vi "PowerEnergyMeterInit.vi"(1 "错误输入（无错误）":errorcluster) -> (0 "错误输出":errorcluster)   [LabVIEW 2012]
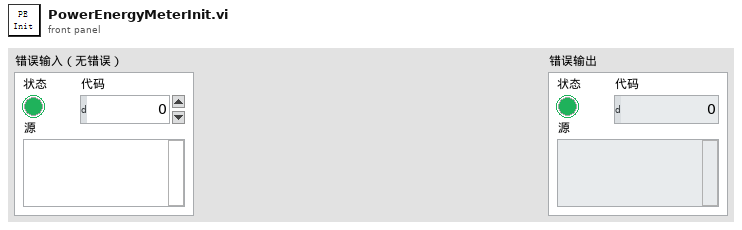
[diagram p1: front panel]
types:
  T1 = typedef "IMAQ Image.ctl" = refnum<image>
  T2 = cluster{"示波器":cluster{"Channel (0:Channel 1)":enum16{"Channel 1", "Channel 2", "Channel 3", "Channel 4"}, "电压范围":dbl, "触发电压":dbl, "时间范围":dbl, " 示波器VISA":refnum<visa-resource-name>}, "光谱仪":cluster{"Channel (0:Channel 1)":enum16{"Channel 1", "Channel 2", "Channel 3", "Channel 4"}, "电压范围":u64, "触发电压":u64, "时间范围":u64}, " 相机1":cluster{"曝光时间":i32, "模拟增益":i32, "控制套接字":i32, "IP 地址":string, " 采集套接字":i32, "  版本号":i32, "ImageData":T1, "  增益最大":i32, "  增益最小":i32, " 曝光最大":i32, " 曝光最小":i32, " 帧速":i32, " 同步切换":i32, "  曝光缩放":i32}, " 偏振仪":cluster{"波长范围":enum16{"可见光", "近红外"}, "电压范围":u64, "触发电压":u64, "时间范围":u64}, " 功率计":cluster{"通道":enum16{"Channel 1", "Channel 2"}, "工作波长":u64, "单位":u64, "时间范围":u64}, "能量计":cluster{"通道":enum16{"Channel 1", "Channel 2"}, "工作波长":u64, "单位":u64, "时间范围":u64}, "电机":cluster{"Channel (0:Channel 1)":enum16{"Channel 1", "Channel 2", "Channel 3", "Channel 4"}, "电压范围":u64, "触发电压":u64, "时间范围":u64}}
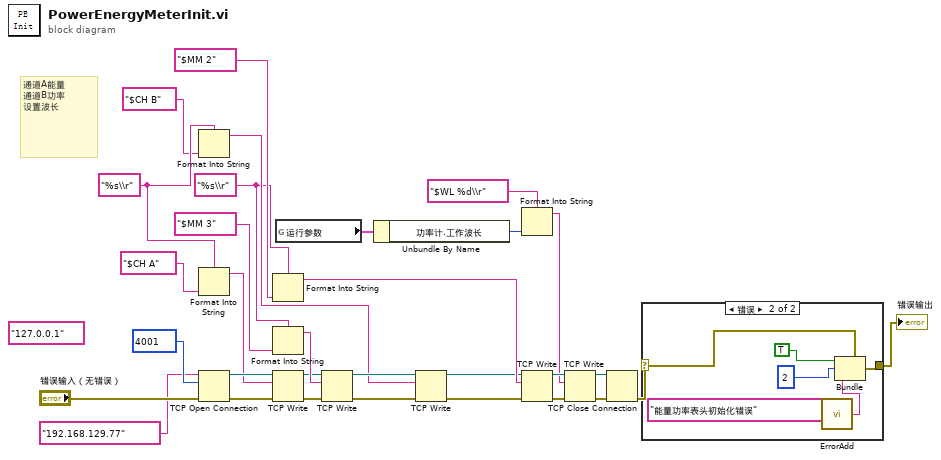
[diagram p0: block diagram]
diagram:
  (unwired) "127.0.0.1" ("地址")
  w20 = "%s\\r" ("格式字符串")
  w12 = "%s\\r" ("格式字符串")
  # "通道A能量\n通道B功率\n设置波长"
  n1 = Format Into String(format string=w20, "$CH B" ("输入 1")) -> (resulting string=w18:string)  [unwired: 2 in, 1 out]
  n2 = Format Into String(format string=w20, "$CH A" ("输入 1")) -> (resulting string=w26:string)  [unwired: 2 in, 1 out]
  n3 = TCP Open Connection(address="192.168.129.77" ("地址"), remote port or service name=u16 4001 ("远程端口或服务名称"), error in (no error)="错误输入（无错误）") -> (connection ID=w27:refnum<k5>, error out=w25:errorcluster)  [unwired: 2 in]
  n4 = Format Into String(format string=w12, "$MM 2" ("输入 1")) -> (resulting string=w15:string)  [unwired: 2 in, 1 out]
  n5 = Format Into String(format string=w12, "$MM 3" ("输入 1")) -> (resulting string=w29:string)  [unwired: 2 in, 1 out]
  n6 = TCP Write(connection ID=w27, data in=w26, error in (no error)=w25) -> (connection ID out=w24:refnum<k5>, error out=w23:errorcluster)  [unwired: 1 in, 1 out]
  n7 = global read "参数.vi" "运行参数"() -> (w10:T2)
  n8 = TCP Write(connection ID=w24, data in=w29, error in (no error)=w23) -> (connection ID out=w21:refnum<k5>, error out=w17:errorcluster)  [unwired: 1 in, 1 out]
  n9 = Unbundle By Name(w10) -> ("功率计.工作波长"=w9:u64)
  n10 = TCP Write(connection ID=w21, data in=w18, error in (no error)=w17) -> (connection ID out=w14:refnum<k5>, error out=w13:errorcluster)  [unwired: 1 in, 1 out]
  n11 = Format Into String(format string="$WL %d\\r" ("格式字符串"), w9) -> (resulting string=w6:string)  [unwired: 2 in, 1 out]
  n12 = TCP Write(connection ID=w14, data in=w15, error in (no error)=w13) -> (connection ID out=w8:refnum<k5>, error out=w7:errorcluster)  [unwired: 1 in, 1 out]
  n13 = TCP Write(connection ID=w8, data in=w6, error in (no error)=w7) -> (connection ID out=w5:refnum<k5>, error out=w4:errorcluster)  [unwired: 1 in, 1 out]
  n14 = TCP Close Connection(connection ID=w5, error in (no error)=w4) -> (error out=w2:errorcluster)  [unwired: 1 in, 1 out]
  n15 = case shown="错误" w2 {
    selector: w2 -> [w32 w34]
    tunnel: [w32 w33] -> w1
    frame No Error {
    }
    frame Error {
      n16 = call "ErrorAdd.vi"("source"="能量功率表头初始化错误") -> ("Errorout Souce"=w35:string)
      n17 = Bundle(cluster=w34, "status"=TRUE, "code"=2, "source"=w35) -> (w33:errorcluster)
    }
  }
  "错误输出" <- w1
